vi "Target4.vi"   [LabVIEW 2025]
uses:
  <vilib>/rvi/DataTransferAndStorage/Container/XNode/niFpgaContainer.xnode
  <vilib>/rvi/interface/RandomDataEmulation/nirviRandomDataFpgaReadWriteTemplate.vi
  <vilib>/rvi/linearAlgebra/MatrixMultiply/XNode/nifxpla_MatrixMultiply.xnode
  <vilib>/rvi/linearAlgebra/MatrixMultiply/simVIs/nifxpla_MatrixMultiply_SimTemplateEinEout.vi
  <vilib>/rvi/linearAlgebra/MatrixMultiply/simVIs/nifxpla_MatrixMultiply_SimTemplateEinVout.vi
  <vilib>/rvi/linearAlgebra/MatrixMultiply/simVIs/nifxpla_MatrixMultiply_SimTemplateVinVout.vi
  <vilib>/rvi/DataTransferAndStorage/Register/Emulation/niFpgaRegisterEmulation.vi
  <vilib>/rvi/DataTransferAndStorage/Register/Emulation/niFpgaRegisterEmulationRefIn.vi
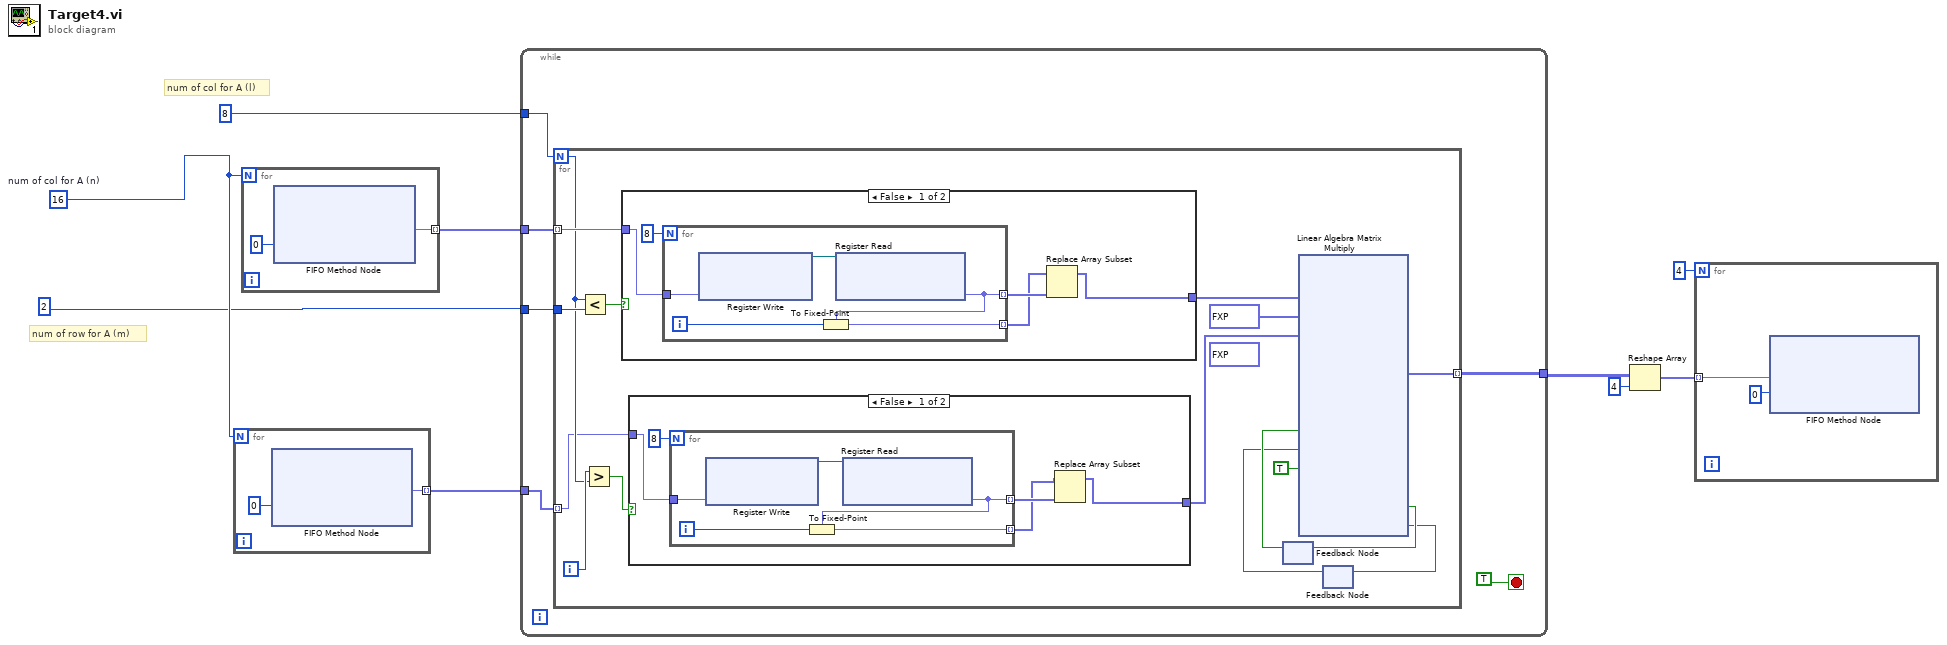
[diagram p0: block diagram]
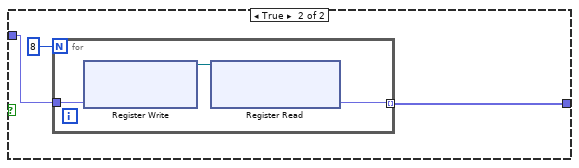
[diagram p2: hidden frame]
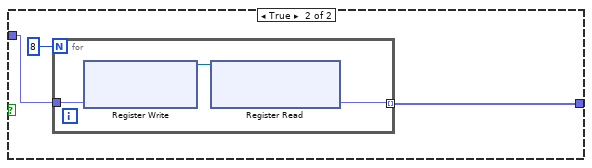
[diagram p3: hidden frame]
diagram:
  w9 = 16  # num of col for A (n)
  # "num of col for A (l)"
  # "num of row for A (m)"
  n1 = for {
    N: w9 -> [_]
    tunnel: [w10] -> w8 mode=indexing
    n2 = xnode ("FIFO Method Node")("Timeout"=0) -> ("Element"=w10:fxp<+/-,32,16>)  [unwired: 1 in, 2 out]
  }
  n3 = for {
    N: w9 -> [_]
    tunnel: [w13] -> w6 mode=indexing
    n4 = xnode ("FIFO Method Node")("Timeout"=0) -> ("Element"=w13:fxp<+/-,32,16>)  [unwired: 1 in, 2 out]
  }
  n5 = while {
    tunnel: w8 -> [w18]
    tunnel: 2 -> [w17]
    tunnel: [w16] -> w4
    tunnel: w6 -> [w15]
    tunnel: 8 -> [w14]
    stop <- TRUE stop-if-true
    n6 = for {
      N: w14 -> [w27]
      tunnel: w18 -> [w24] mode=indexing
      tunnel: w17 -> [w33]
      tunnel: [w31] -> w16 mode=indexing
      tunnel: w15 -> [w30] mode=indexing
      i -> [w28]
      (unwired) fxp<+/-,32,16>[] [0.0, 0.0] ("bi")
      n7 = Less?(x=w27, y=w33) -> (x < y?=w34:bool)
      n8 = Greater?(x=w28, y=w27) -> (0:w25:bool)
      n9 = case shown="False" w34 {
        tunnel: [w54 w63] -> w32
        tunnel: w30 -> [w55 w62]
        frame False {
          n10 = for {
            N: 8 -> [_]
            tunnel: w55 -> [w61]
            tunnel: [w57] -> w53 mode=indexing
            tunnel: [w58] -> w52 mode=indexing
            i -> [w59]
            n11 = xnode "Register Write"("Data"=w61) -> ("Register Out"=w60:refnum<k21>)  [unwired: 1 in]
            n12 = xnode "Register Read"("Register In"=w60) -> ("Data"=w57:fxp<+/-,32,16>)  [unwired: 1 out]
            n13 = To Fixed-Point(fixed-point type=w57, number=w59) -> (fixed-point=w58:fxp<+/-,32,16>)
          }
          n14 = Replace Array Subset(array=w52, new element=w53) -> (w54:fxp<+/-,32,16>[])  [unwired: 1 in]
        }
        frame True {
          n15 = for {
            N: 8 -> [_]
            tunnel: [w66] -> w63 mode=indexing
            tunnel: w62 -> [w65]
            n16 = xnode "Register Write"("Data"=w65) -> ("Register Out"=w67:refnum<k21>)  [unwired: 1 in]
            n17 = xnode "Register Read"("Register In"=w67) -> ("Data"=w66:fxp<+/-,32,16>)  [unwired: 1 out]
          }
        }
      }
      n18 = case shown="False" w25 {
        tunnel: [w38 w47] -> w26
        tunnel: w24 -> [w39 w46]
        frame False {
          n19 = for {
            N: 8 -> [_]
            tunnel: w39 -> [w45]
            tunnel: [w41] -> w37 mode=indexing
            tunnel: [w42] -> w36 mode=indexing
            i -> [w43]
            n20 = xnode "Register Write"("Data"=w45) -> ("Register Out"=w44:refnum<k21>)  [unwired: 1 in]
            n21 = xnode "Register Read"("Register In"=w44) -> ("Data"=w41:fxp<+/-,32,16>)  [unwired: 1 out]
            n22 = To Fixed-Point(fixed-point type=w41, number=w43) -> (fixed-point=w42:fxp<+/-,32,16>)
          }
          n23 = Replace Array Subset(array=w36, new element=w37) -> (w38:fxp<+/-,32,16>[])  [unwired: 1 in]
        }
        frame True {
          n24 = for {
            N: 8 -> [_]
            tunnel: [w50] -> w47 mode=indexing
            tunnel: w46 -> [w49]
            n25 = xnode "Register Write"("Data"=w49) -> ("Register Out"=w51:refnum<k21>)  [unwired: 1 in]
            n26 = xnode "Register Read"("Register In"=w51) -> ("Data"=w50:fxp<+/-,32,16>)  [unwired: 1 out]
          }
        }
      }
      n27 = feedback #1() -> (w22:bool)  [unwired: 1 in]
      n28 = feedback #2() -> (w20:bool)  [unwired: 1 in]
      n29 = xnode ("Linear Algebra Matrix Multiply")("ar"=w32, "ai"=fxp<+/-,32,16>[] [0.0, 0.0, 0.0, 0.0, 0.0, 0.0, 0.0, 0.0], "br"=w26, "a valid"=w22, "b valid"=w20, "ready for output (T)"=TRUE) -> ("cr"=w31:fxp<+/-,64,35>[], "ready for a"=w23:bool, "ready for b"=w21:bool)  [unwired: 1 in, 3 out]
      n30 = feedback-in #1(w23) -> ()
      n31 = feedback-in #2(w21) -> ()
    }
  }
  n32 = Reshape Array(w4, 4 ("dimension size")) -> (w3:fxp<+/-,64,35>[])
  n33 = for {
    N: 4 -> [_]
    tunnel: w3 -> [w69] mode=indexing
    n34 = xnode ("FIFO Method Node")("Element"=w69, "Timeout"=0) -> ()  [unwired: 1 in, 2 out]
  }
